vi "Gen Stage 3 Resolve gRPC Dependencies.vi"(7 "Staus":refnum<vi>, 8 "error in":errorcluster, 9 "Proto Names":T1, 10 "New Subname":string, 11 "Template Project Path":path) -> (0 "error out":errorcluster)   [LabVIEW 2021, in "Plugin Generator.lvlib"]
uses:
  Plugin Generator.lvlib
  Typedef/Proto Names.ctl
  <vilib>/CIF Foundation/CIF LabVIEW Scripting/LV Scripting/LV Scripting Utilities.lvlib
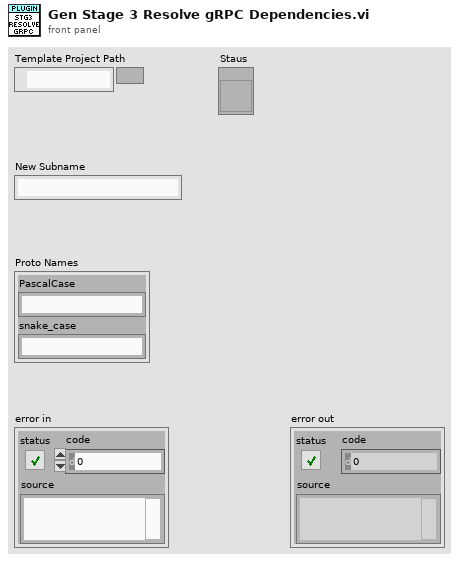
[diagram p1: front panel]
types:
  T1 = typedef "Plugin Generator.lvlib/Proto Names.ctl" = cluster{"PascalCase":string, "snake_case":string}
  T2 = typedef "LV Scripting Utilities.lvlib/Target References.ctl" = cluster{"Target Reference":refnum<vi>, "VI References":refnum<vi>[], "Library References":refnum<vi>[], "Build References":refnum<vi>[]}
  T3 = typedef "LV Scripting Utilities.lvlib/Library Map.ctl" = map{string, refnum<vi>}
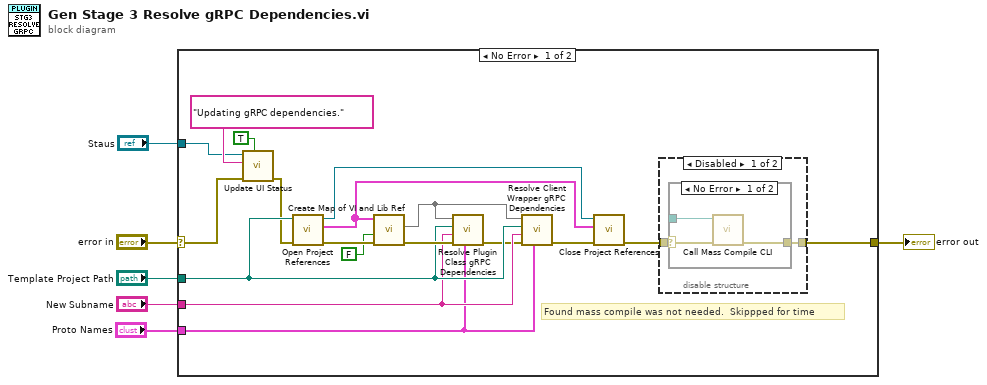
[diagram p0: block diagram]
diagram:
  n1 = case shown="No Error" "error in" {
    selector: "error in" -> [w9 w32]
    tunnel: [w24 w32] -> w6
    tunnel: "Proto Names" -> [w14 _]
    tunnel: "Template Project Path" -> [w17 _]
    tunnel: "New Subname" -> [w15 _]
    tunnel: "Staus" -> [w10 _]
    frame No Error {
      # "Found mass compile was not needed.  Skippped for time"
      n2 = call "Update UI Status.vi"("Previous Complete"=TRUE, "error in"=w9, "Status to Display"="Updating gRPC dependencies." ("To display"), "String in"=w10) -> ("error out"=w8:errorcluster)  [unwired: 7 in]
      n3 = call <vilib>:"Open Project References.vi"("error in"=w8, "Project Path"=w17) -> ("error out"=w22:errorcluster, "VI, Library, and Build References"=w20:T2[], "Project Reference"=w21:refnum<vi>)  [unwired: 7 in]
      n4 = call <vilib>:"Create Map of VI and Lib Ref.vi"("error in"=w22, "RT Target"=FALSE, "VI, Library, and Build References"=w20) -> ("error out"=w23:errorcluster, "Library Map"=w16:T3)  [unwired: 5 in, 2 out]
      n5 = call "Resolve Plugin Class gRPC Dependencies.vi"("Proto Names"=w14, "error in"=w23, "New Subname"=w15, "Template Project Path"=w17, "Map - LibRef"=w16) -> ("error out"=w13:errorcluster)  [unwired: 6 in]
      n6 = call "Resolve Client Wrapper gRPC Dependencies.vi"("Proto Names"=w14, "error in"=w13, "New Subname"=w15, "Template Project Path"=w17, "Map - LibRef"=w16) -> ("error out"=w12:errorcluster)  [unwired: 6 in]
      n7 = call <vilib>:"Close Project References.vi"("error in"=w12, "VI, Library, and Build References"=w20, "Project Reference"=w21) -> ("error out"=w18:errorcluster)  [unwired: 8 in]
      n8 = disable-structure shown="Disabled" {
        disable-tunnel: [w26 w31] -> w24
        disable-tunnel: w18 -> [w25 w31]
        frame Disabled {
          n9 = case shown="No Error" w25 {
            selector: w25 -> [w28 w30]
            tunnel: [w27 w30] -> w26
            tunnel: _ -> [w29 _]
            frame No Error {
              n10 = call <vilib>:"Call Mass Compile CLI.vi"("error in"=w28, "Directory"=w29) -> ("error out"=w27:errorcluster)  [unwired: 9 in]
            }
            frame Error {
            }
          }
        }
        frame Enabled {
        }
      }
    }
    frame Error {
    }
  }
  "error out" <- w6
